vi "Col_distance_GPS(Subvi).vi"(8 "2_위도":dbl, 9 "1_위도":dbl, 10 "Delta_lon":dbl, 11 "Delta_lat":dbl) -> (3 "distance[m]":dbl)   [LabVIEW 2024]
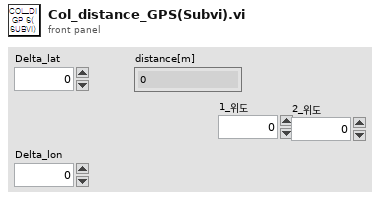
[diagram p1: front panel]
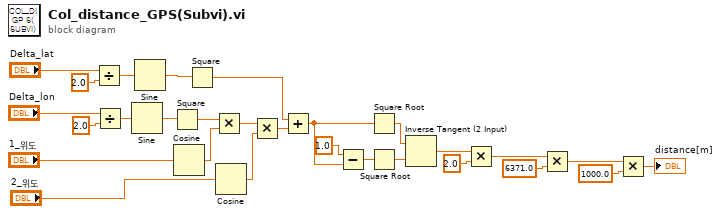
[diagram p0: block diagram]
diagram:
  n1 = Divide(x="Delta_lat", y=2.0) -> (x/y=w4:dbl)
  n2 = Divide(x="Delta_lon", y=2.0) -> (x/y=w7:dbl)
  n3 = Sine(x=w7) -> (sin(x)=w6:dbl)
  n4 = Sine(x=w4) -> (sin(x)=w5:dbl)
  n5 = Square(x=w6) -> (x^2=w9:dbl)
  n6 = Cosine(x="1_위도") -> (cos(x)=w10:dbl)
  n7 = Square(x=w5) -> (x^2=w20:dbl)
  n8 = Multiply(x=w9, y=w10) -> (x*y=w11:dbl)
  n9 = Cosine(x="2_위도") -> (cos(x)=w12:dbl)
  n10 = Multiply(x=w11, y=w12) -> (x*y=w19:dbl)
  n11 = Add(x=w20, y=w19) -> (x+y=w21:dbl)
  n12 = Subtract(x=1.0, y=w21) -> (x-y=w14:dbl)
  n13 = Square Root(x=w21) -> (sqrt(x)=w22:dbl)
  n14 = Square Root(x=w14) -> (sqrt(x)=w23:dbl)
  n15 = Inverse Tangent (2 Input)(1:w23, 2:w22) -> (0:w16:dbl)
  n16 = Multiply(x=w16, y=2.0) -> (x*y=w18:dbl)
  n17 = Multiply(x=w18, y=6371.0) -> (x*y=w24:dbl)
  n18 = Multiply(x=w24, y=1000.0) -> (x*y=→"distance[m]":dbl)
